vi "get results reporter.vi"(11 "task in":refnum<class "task.lvclass">) -> (2 "results reporter":refnum<class "results reporter.lvclass">, 3 "task out":refnum<class "task.lvclass">)   [LabVIEW 2013, in "task.lvclass"]
uses:
  task.lvclass
  results reporter/results reporter.lvclass
  task.lvclass/task.ctl
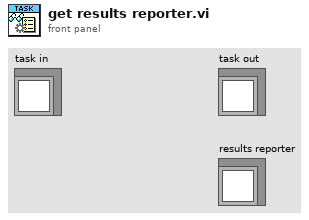
[diagram p1: front panel]
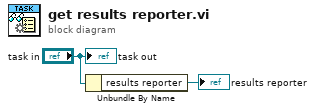
[diagram p0: block diagram]
diagram:
  n1 = Unbundle By Name("task in") -> ("results reporter"=→"results reporter":refnum<class "results reporter.lvclass">)
  "task out" <- "task in"
